vi "Parse BTI MSGACT.vi"(11 "msgact":u16 format="%016b") -> (0 "specific errors":T1, 1 "receiving error":bool, 2 "hit":bool, 3 "hardware channel":u8, 4 "speed":enum16{"Low", "High"}(ring))   [LabVIEW 2020, in "Ballard ARINC 429 Engine.lvlib" / "Custom Device.lvlib"]
uses:
  Custom Device.lvlib
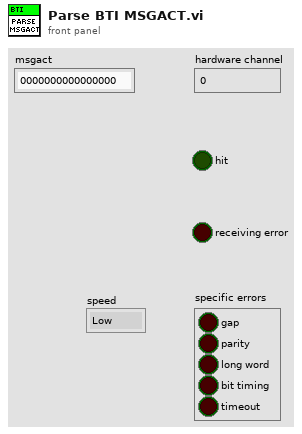
[diagram p1: front panel]
types:
  T1 = cluster{"gap":bool, "parity":bool, "long word":bool, "bit timing":bool, "timeout":bool}
  T2 = cluster{"[0]":bool, "[1]":bool, "[2]":bool, "[3]":bool, "[4]":bool}
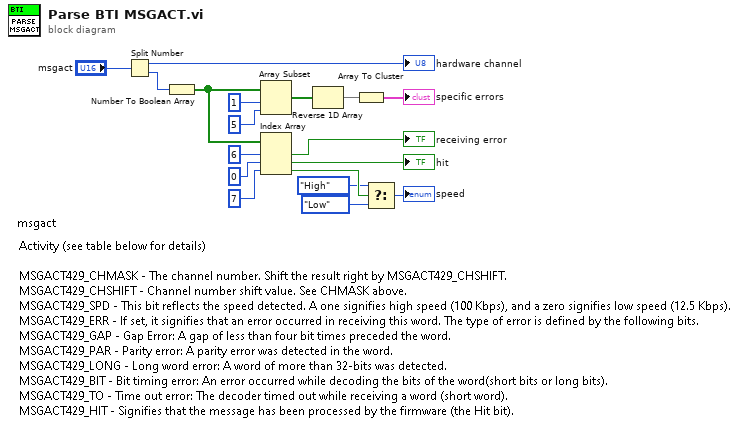
[diagram p0: block diagram]
diagram:
  n1 = Split Number(x="msgact") -> (hi(x)=→"hardware channel":u8, lo(x)=w16:u8)
  n2 = Number To Boolean Array(number=w16) -> (Boolean array=w15:bool[])
  n3 = Array Subset(array=w15, index=1, length=5) -> (w12:bool[])
  n4 = Index Array(array=w15, index #1=6 ("index"), index #2=0 ("index"), index #3=7 ("index")) -> (element #1=→"receiving error":bool, element #2=→"hit":bool, element #3=w4:bool)
  n5 = Reverse 1D Array(array=w12) -> (reversed array=w11:bool[])
  n6 = Array To Cluster(array=w11) -> (cluster=→"specific errors":T2)
  n7 = Select(t=enum16{"Low", "High"}."High" ("speed"), s=w4, f=enum16{"Low", "High"}."Low" ("speed")) -> (s? t:f=→"speed":enum16{"Low", "High"})
